vi "face rotate.vi"(6 "rotation directon":T1, 8 "error in (no error)":errorcluster, 11 "face in":T2) -> (0 "error out":errorcluster, 3 "face out":T2)   [LabVIEW 2011]
uses:
  Typedef/face.ctl
  Typedef/face rotate direction.ctl
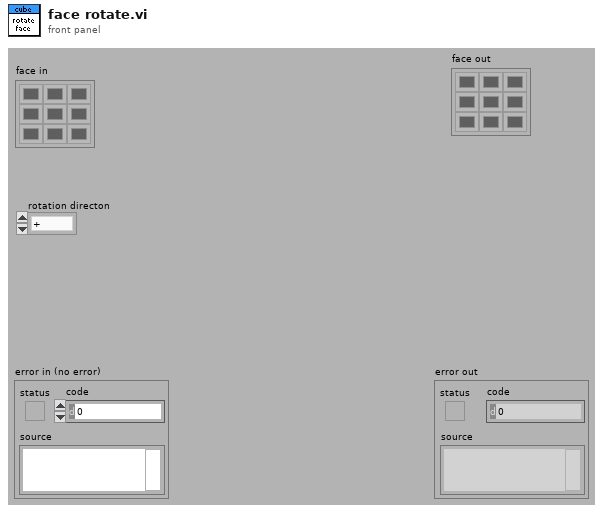
[diagram p1: front panel]
types:
  T1 = typedef "face rotate direction.ctl" = enum16{"+", "-"}
  T2 = typedef "face.ctl" = u32[][]
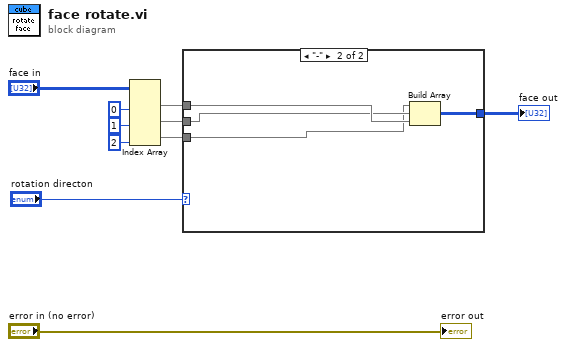
[diagram p0: block diagram]
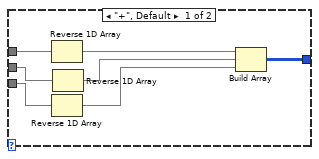
[diagram p2: hidden frame]
diagram:
  n1 = Index Array(array="face in", index (col) #1=0 ("disabled index (col)"), index (col) #2=1 ("index (col)"), index (col) #3=2 ("index (col)")) -> (element #1=w8:u32[], element #2=w5:u32[], element #3=w4:u32[])  [unwired: 3 in]
  n2 = case shown="\"-\"" "rotation directon" {
    tunnel: w8 -> [w17 w20]
    tunnel: w5 -> [w15 w19]
    tunnel: w4 -> [w14 w18]
    tunnel: [w11 w21] -> w3
    frame "+", Default {
      n3 = Reverse 1D Array(array=w17) -> (reversed array=w16:u32[])
      n4 = Reverse 1D Array(array=w14) -> (reversed array=w12:u32[])
      n5 = Reverse 1D Array(array=w15) -> (reversed array=w13:u32[])
      n6 = Build Array(w16, w13, w12) -> (w11:u32[][])
    }
    frame "-" {
      n7 = Build Array(w18, w19, w20) -> (w21:u32[][])
    }
  }
  "face out" <- w3
  "error out" <- "error in (no error)"
